vi "RemoveObserver.vi"(8 "error in (no error)":errorcluster, 10 "ObserverNotifierReference":refnum<notifier>, 11 "Observable in":refnum<class "Observable.lvclass">) -> (0 "error out":errorcluster, 3 "Observable out":refnum<class "Observable.lvclass">)   [LabVIEW 2013, in "Observable.lvclass"]
uses:
  Observable.lvclass
  Observable.lvclass/Observable.ctl
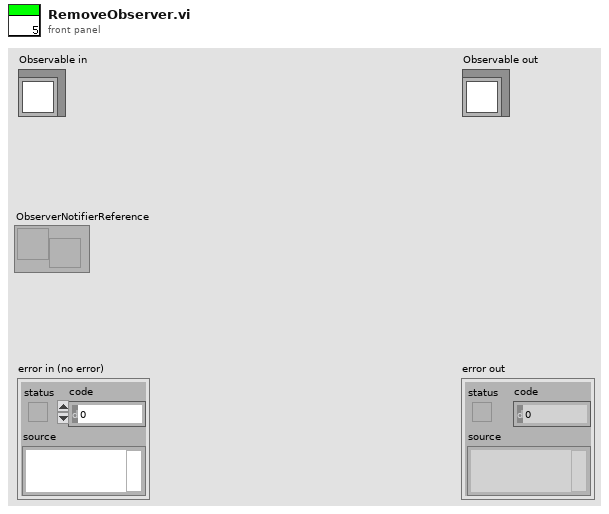
[diagram p1: front panel]
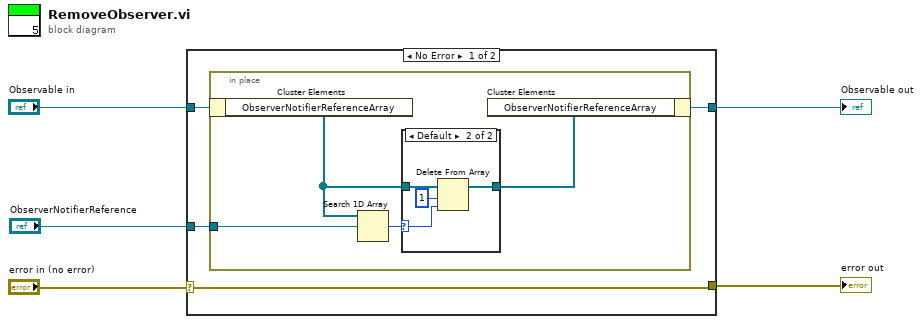
[diagram p0: block diagram]
diagram:
  n1 = case shown="No Error" "error in (no error)" {
    selector: "error in (no error)" -> [w6 w20]
    tunnel: [w6 w20] -> w4
    tunnel: [w8 w19] -> w2
    tunnel: "Observable in" -> [w9 w19]
    tunnel: "ObserverNotifierReference" -> [w7 _]
    frame No Error {
      n2 = in-place {
        in-place-border: w7 -> [w10]
        n3 = in-place-cluster #1(w9) -> ("ObserverNotifierReferenceArray"=w11:refnum<notifier>[])
        n4 = Search 1D Array(1D array=w11, element=w10) -> (index of element=w12:i32)  [unwired: 1 in]
        n5 = case shown="Default" w12 {
          selector: w12 -> [_ w16]
          tunnel: w11 -> [w14 w18]
          tunnel: [w14 w15] -> w13
          frame -1 {
          }
          frame Default {
            n6 = Delete From Array(array=w18, length=1, index=w16) -> (array with subset deleted=w15:refnum<notifier>[])  [unwired: 1 out]
          }
        }
        n7 = in-place-cluster #1("ObserverNotifierReferenceArray"=w13) -> (w8:refnum<class "Observable.lvclass">)
      }
    }
    frame Error {
    }
  }
  "error out" <- w4
  "Observable out" <- w2
